vi "readFrame.vi"(8 "error in (no error)":errorcluster, 10 "RGB32 Image in":T1, 11 "TCP Network Connection in":refnum<k5>) -> (0 "error out":errorcluster, 2 "Image out":T1(plugin-control), 3 "TCP Network Connection out":refnum<k5>)   [LabVIEW 2016]
uses:
  <vilib>/vision/Image Controls.llb/IMAQ Image.ctl
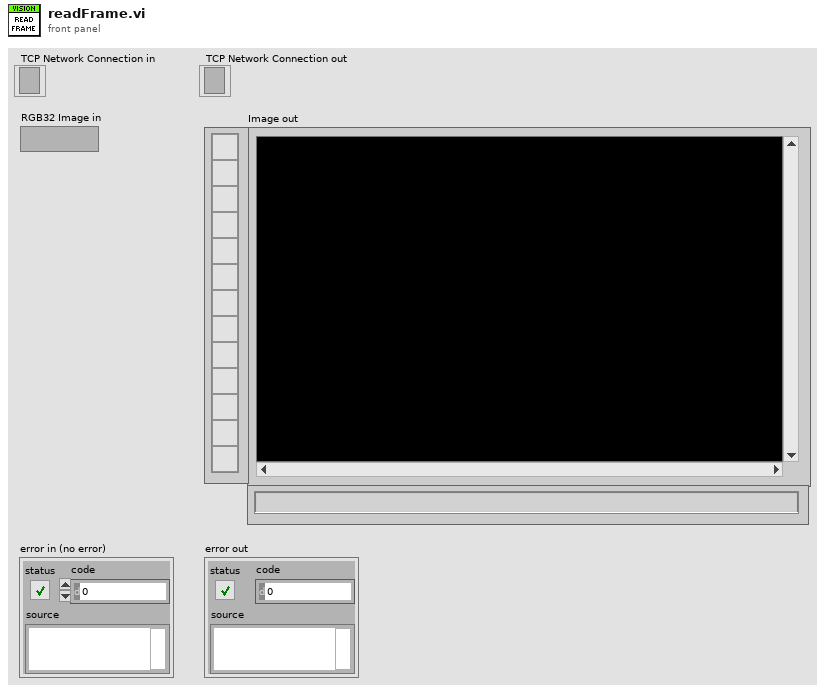
[diagram p1: front panel]
types:
  T1 = typedef "IMAQ Image.ctl" = refnum<image>
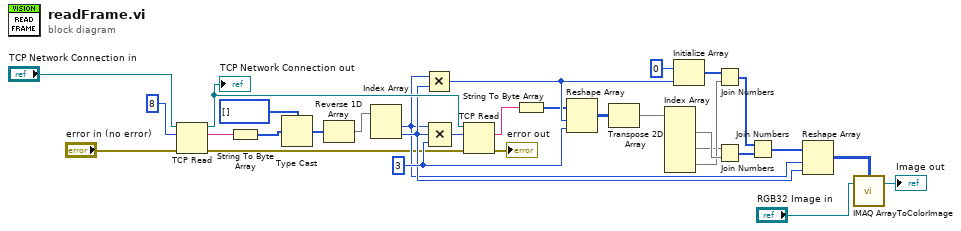
[diagram p0: block diagram]
diagram:
  w11 = 3 ("value")
  n1 = TCP Read(connection ID="TCP Network Connection in", bytes to read=8, error in (no error)="error in (no error)") -> (connection ID out=w31:refnum<k5>, data out=w2:string, error out=w6:errorcluster)  [unwired: 2 in]
  "TCP Network Connection out" <- w31
  n2 = String To Byte Array(string=w2) -> (unsigned byte array=w3:u8[])
  n3 = Type Cast(type=i32[] [], x=w3) -> (*(type *) &x=w26:i32[])
  n4 = Reverse 1D Array(array=w26) -> (reversed array=w27:i32[])
  n5 = Index Array(array=w27) -> (element #1=w9:i32, element #2=w10:i32)  [unwired: 2 in]
  n6 = Multiply(x=w9, y=w10) -> (x*y=w19:i32)
  n7 = Compound Arithmetic op=MULTIPLY(w9, w10, w11) -> (w5:i32)
  n8 = TCP Read(connection ID=w31, bytes to read=w5, error in (no error)=w6) -> (data out=w7:string, error out=→"error out":errorcluster)  [unwired: 2 in, 1 out]
  n9 = String To Byte Array(string=w7) -> (unsigned byte array=w12:u8[])
  n10 = Reshape Array(w12, w19, w11) -> (w24:u8[][])
  n11 = Transpose 2D Array(2D array=w24) -> (transposed array=w25:u8[][])
  n12 = Index Array(array=w25) -> (element #1=w23:u8[], element #2=w13:u8[], element #3=w22:u8[])  [unwired: 6 in]
  n13 = Initialize Array(u8 0, w19) -> (w21:u8[])
  n14 = Join Numbers(hi=w21, lo=w22) -> ((hi.lo)=w15:u16[])
  n15 = Join Numbers(hi=w13, lo=w23) -> ((hi.lo)=w14:u16[])
  n16 = Join Numbers(hi=w15, lo=w14) -> ((hi.lo)=w8:u32[])
  n17 = Reshape Array(w8, w9, w10) -> (w28:u32[][])
  n18 = call "IMAQ ArrayToColorImage"("Image Pixels (U32)"=w28, "Image"="RGB32 Image in") -> ("Image Out"=→"Image out":T1)  [unwired: 3 in, 1 out]
